vi "RemoveBackspace.vi"(10 "read buffer":string, 11 "Console In":string) -> (3 "String":string)   [LabVIEW 2019]
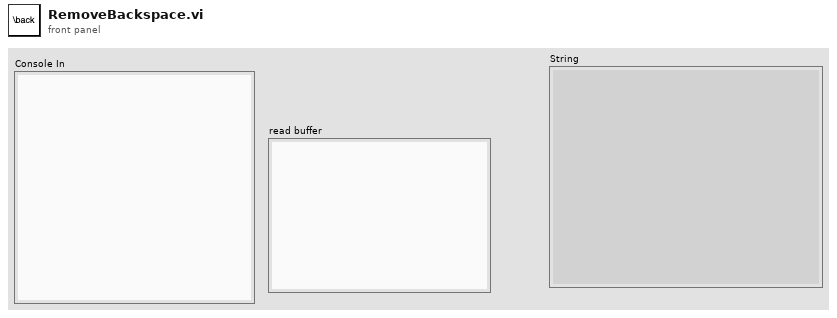
[diagram p1: front panel]
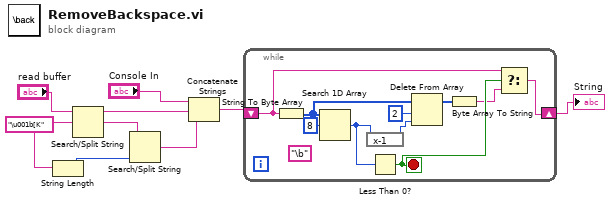
[diagram p0: block diagram]
diagram:
  w3 = "\u001b[K"
  n1 = String Length(string=w3) -> (length=w2:i32)
  n2 = Search/Split String(string="read buffer", search string/char (-)=w3) -> (substring before match=w8:string, match + rest of string=w4:string)  [unwired: 1 in, 1 out]
  n3 = Search/Split String(string=w4, offset (0)=w2) -> (match + rest of string=w1:string)  [unwired: 1 in, 2 out]
  n4 = Concatenate Strings("Console In", w8, w1) -> (w6:string)
  n5 = while {
    shift-right: [w10] -> w5
    shift-left: w6 -> [w12]
    stop <- w13 stop-if-true
    (unwired) "\b"
    n6 = String To Byte Array(string=w12) -> (unsigned byte array=w18:u8[])
    n7 = Search 1D Array(1D array=w18, element=u8 8) -> (index of element=w14:i32)  [unwired: 1 in]
    n8 = expression code="x-1"(w14) -> (w16:i32)
    n9 = Less Than 0?(x=w14) -> (x < 0?=w13:bool)
    n10 = Delete From Array(array=w18, length=2, index=w16) -> (array with subset deleted=w15:u8[])  [unwired: 1 out]
    n11 = Byte Array To String(unsigned byte array=w15) -> (string=w11:string)
    n12 = Select(t=w12, s=w13, f=w11) -> (s? t:f=w10:string)
  }
  "String" <- w5
